vi "get Zoom.vi"(11 "Camera in":refnum<class "Camera.lvclass">) -> (3 "Zoom Level":sgl)   [LabVIEW 2021, in "Camera.lvclass"]
uses:
  Camera.lvclass
  Camera.lvclass/Camera.ctl
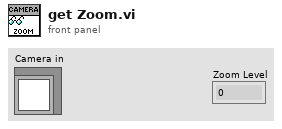
[diagram p1: front panel]
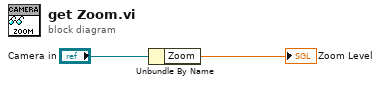
[diagram p0: block diagram]
diagram:
  n1 = Unbundle By Name("Camera in") -> ("Zoom"=→"Zoom Level":sgl)
